vi "Set Sciscan Dynamics.vi"(8 "error in":errorcluster, 10 "Fast":bool, 11 "GFG Refnum":refnum<vi>) -> (0 "error out":errorcluster, 3 "GFG Refnum Out":refnum<vi>)   [LabVIEW 2012, in "Sciscan Scope Daemon.lvlib"]
uses:
  Sciscan Scope Daemon.lvlib
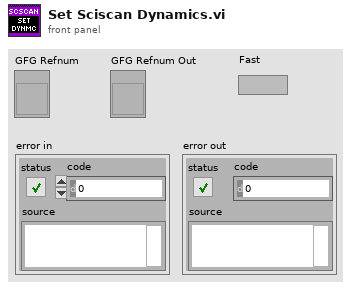
[diagram p1: front panel]
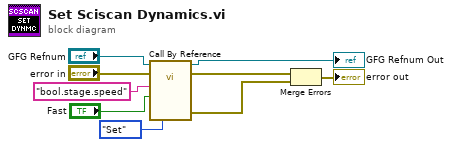
[diagram p0: block diagram]
diagram:
  n1 = call-by-ref "?"(reference="GFG Refnum", error in="error in", "Variable Name in"="bool.stage.speed", "Variant in"="Fast", "Action"=enum16{"Init", "Set", "Get"}."Set") -> (reference out=→"GFG Refnum Out":refnum<vi>, error out=w8:errorcluster, 19:"error out"=w7:errorcluster)  [unwired: 10 in, 6 out]
  n2 = Merge Errors(w8, w7) -> (→"error out":errorcluster)
